vi "Initialize Subpanel UI.vi"(8 "error in (no error)":errorcluster, 11 "Plugin in":refnum<class "Generic Plugin.lvclass">) -> (0 "error out":errorcluster, 2 "Subpanel UI Reference":refnum<vi>, 3 "Plugin out":refnum<class "Generic Plugin.lvclass">)   [LabVIEW 2020, in "Generic Plugin.lvclass"]
doc: "Initialize the subpanel UI VI reference and message queue inside the class, also giving the subpanel UI the correct message queue for further communication."
uses:
  Generic Plugin.lvclass
  Generic Plugin.lvclass/Generic Plugin.ctl
  Sub VIs/Message Queue/test Message Queue.lvlib
  Sub VIs/Message Queue/Enqueue Message (Single).vi
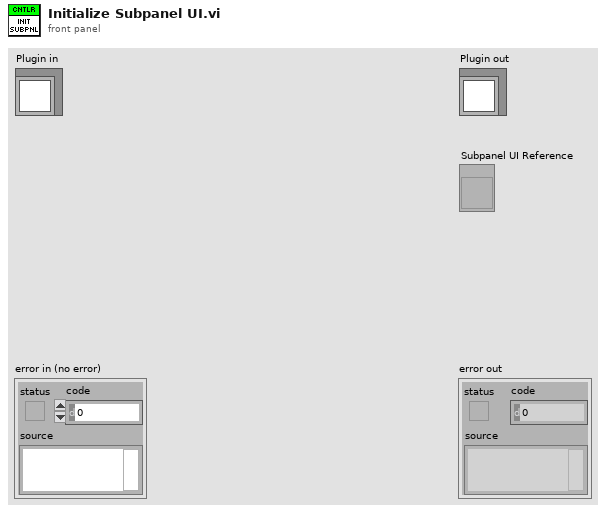
[diagram p1: front panel]
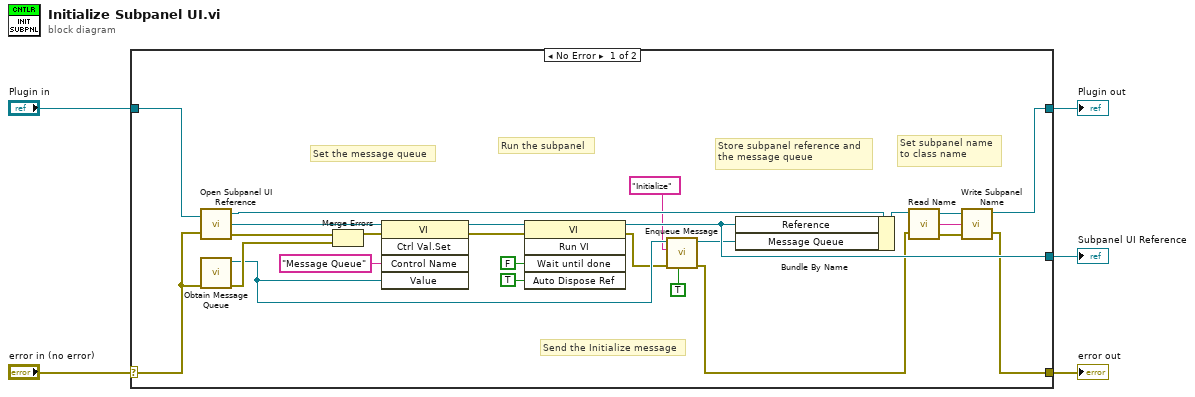
[diagram p0: block diagram]
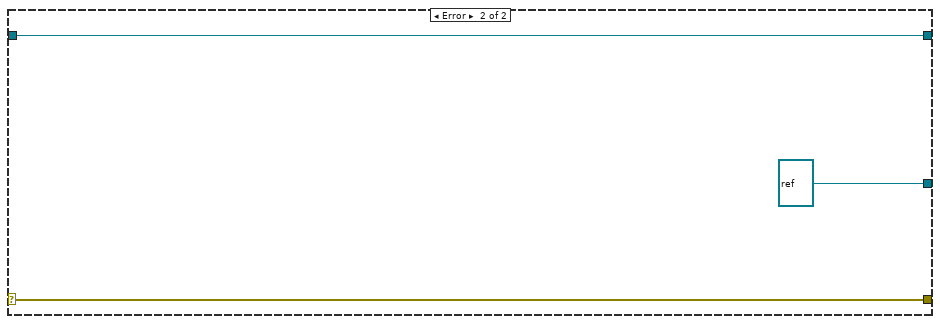
[diagram p2: hidden frame]
diagram:
  n1 = case shown="No Error" "error in (no error)" {
    selector: "error in (no error)" -> [w26 w33]
    tunnel: [w6 w33] -> w4
    tunnel: [w11 w32] -> w2
    tunnel: "Plugin in" -> [w29 w32]
    tunnel: [w16 refnum<vi> refnum ("vi reference")] -> w1
    frame No Error {
      # "Set subpanel name\nto class name"
      # "Send the Initialize message"
      # "Store subpanel reference and\nthe message queue"
      # "Run the subpanel"
      # "Set the message queue"
      n2 = call "Open Subpanel UI Reference.vi"("Controller in"=w29, "error in (no error)"=w26) -> ("Controller out"=w27:refnum<class "Generic Plugin.lvclass">, "vi reference"=w28:refnum<vi>, "error out"=w24:errorcluster)
      n3 = call "Obtain Message Queue.vi"("error in (no error)"=w26) -> ("error out"=w22:errorcluster, "Message Queue"=w17:refnum<queue>)  [unwired: 9 in]
      n4 = Merge Errors(w24, w22) -> (w23:errorcluster)
      n5 = invoke class="VI" method="Ctrl Val.Set"(reference=w28, error in=w23, "Control Name"="Message Queue", "Value"=w17) -> (reference out=w25:refnum<vi>, error out=w20:errorcluster)  [unwired: 1 in, 3 out]
      n6 = invoke class="VI" method="Run VI"(reference=w25, error in=w20, "Wait until done"=FALSE ("Wait Until Done"), "Auto Dispose Ref"=TRUE ("Auto Dispose Reference")) -> (reference out=w16:refnum<vi>, error out=w14:errorcluster)  [unwired: 1 in, 3 out]
      n7 = call-poly "Enqueue Message.vi"("Priority Message? (F)"=TRUE, "error in (no error)"=w14, "Message"="Initialize", "Message Queue"=w17) -> ("error out"=w7:errorcluster, "dup Message Queue"=w15:refnum<queue>)  [unwired: 6 in]
      n8 = Bundle By Name(cluster=w27, "Reference"=w16, "Message Queue"=w15) -> (w30:refnum<class "Generic Plugin.lvclass">)
      n9 = call "Read Name.vi"("controller in"=w30, "error in (no error)"=w7) -> ("controller out"=w10:refnum<class "Generic Plugin.lvclass">, "Name"=w9:string, "error out"=w8:errorcluster)
      n10 = call "Write Subpanel Name.vi"("error in (no error)"=w8, "Name"=w9, "Controller in"=w10) -> ("error out"=w6:errorcluster, "Controller out"=w11:refnum<class "Generic Plugin.lvclass">)
    }
    frame Error {
    }
  }
  "error out" <- w4
  "Plugin out" <- w2
  "Subpanel UI Reference" <- w1
